vi "Is_Active_Call.vi"(5 "Enum":T1(ring), 6 "error in (no error)":errorcluster, 7 "Floor":i32, 8 "Elevator in":T3, 9 "Elevator Fleet in":T2) -> (0 "error out":errorcluster, 1 "Active Call?":bool, 2 "Elevator out":T3, 3 "Elevator Fleet out":T2)   [LabVIEW 2026]
uses:
  Controls/Elevator_Status.ctl
  Controls/Door_Status_Enum.ctl
  Controls/Occupy_Status.ctl
  Controls/Floor_Status.ctl
  Controls/Motion_Status_Enum.ctl
  Controls/Car_Calls_Status.ctl
  Controls/Hall_Calls_Status.ctl
  Controls/Elevator_Fleet.ctl
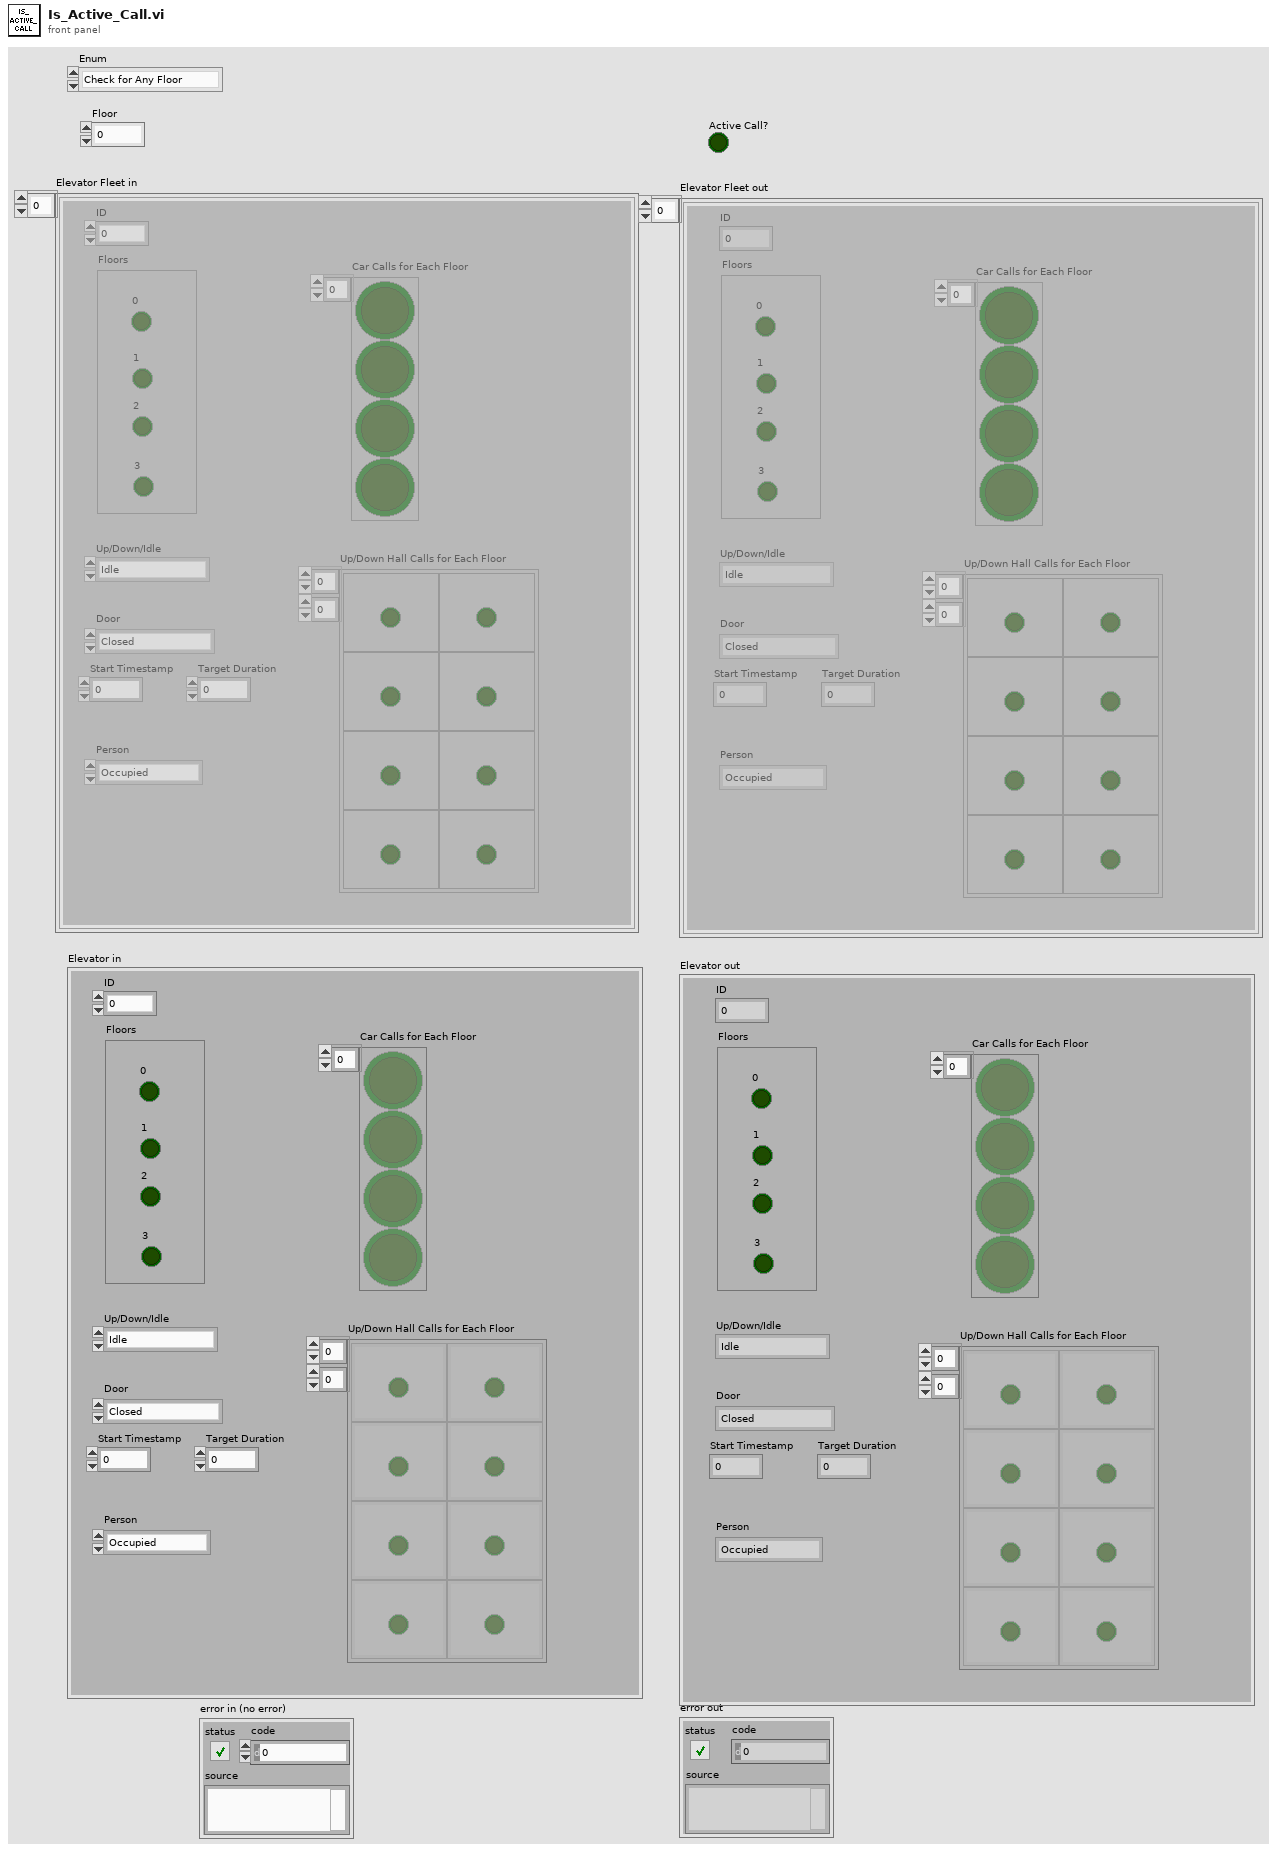
[diagram p1: front panel]
types:
  T1 = enum16{"Check for Any Floor", "Check for Specific Floor"}
  T2 = typedef "Elevator_Fleet.ctl" = T3[]
  T3 = typedef "Elevator_Status.ctl" = cluster{"Door":T4, "Person":T5, "Floors":T6, "Up/Down/Idle":T7, "Car Calls for Each Floor":T8, "Up/Down Hall Calls for Each Floor":T9, "ID":i32, "Start Timestamp":u32, "Target Duration":dbl}
  T4 = typedef "Door_Status_Enum.ctl" = enum16{"Closed", "Open", "Opening", "Closing"}
  T5 = typedef "Occupy_Status.ctl" = enum16{"Occupied", "Empty"}
  T6 = typedef "Floor_Status.ctl" = cluster{"0":bool, "1":bool, "2":bool, "3":bool}
  T7 = typedef "Motion_Status_Enum.ctl" = enum16{"Idle", "Up", "Down"}
  T8 = typedef "Car_Calls_Status.ctl" = bool[]
  T9 = typedef "Hall_Calls_Status.ctl" = cluster{bool}[][]
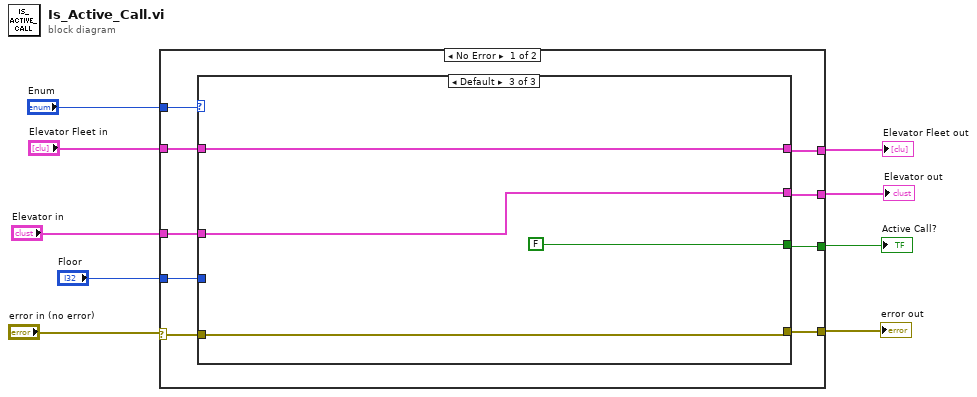
[diagram p0: block diagram]
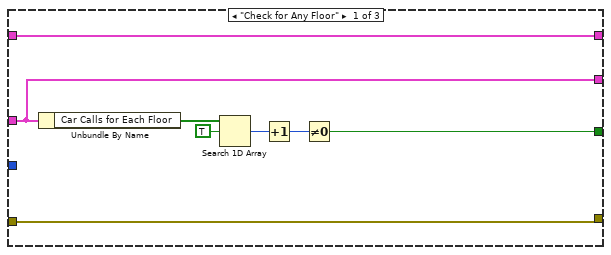
[diagram p2: hidden frame]
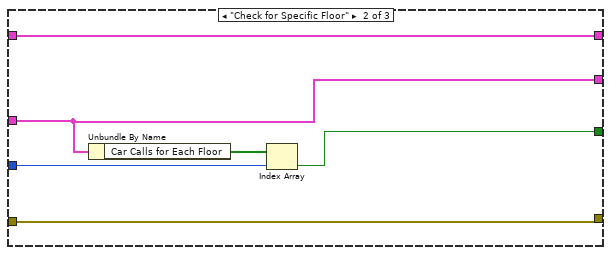
[diagram p3: hidden frame]
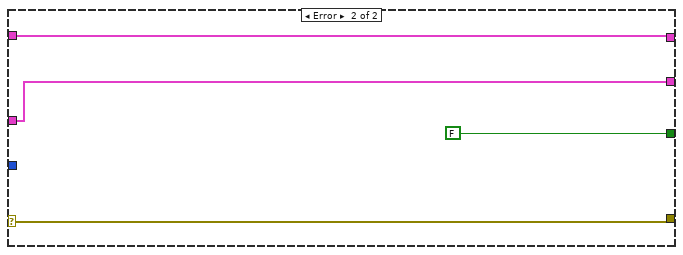
[diagram p4: hidden frame]
diagram:
  n1 = case shown="No Error" "error in (no error)" {
    selector: "error in (no error)" -> [w12 w38]
    tunnel: "Elevator in" -> [w18 w39]
    tunnel: [w17 FALSE] -> w8
    tunnel: [w16 w39] -> w7
    tunnel: "Elevator Fleet in" -> [w15 w40]
    tunnel: [w14 w40] -> w5
    tunnel: "Enum" -> [w13 _]
    tunnel: [w11 w38] -> w2
    tunnel: "Floor" -> [w10 _]
    frame No Error {
      n2 = case shown="Default" w13 {
        tunnel: w18 -> [w21 w30 w35]
        tunnel: [w22 w27 FALSE] -> w17
        tunnel: [w21 w30 w35] -> w16
        tunnel: w15 -> [w20 w31 w36]
        tunnel: [w20 w31 w36] -> w14
        tunnel: [w19 w32 w33] -> w11
        tunnel: w12 -> [w19 w32 w33]
        tunnel: w10 -> [_ w28 _]
        frame "Check for Any Floor" {
          n3 = Unbundle By Name(w21) -> ("Car Calls for Each Floor"=w26:T8)
          n4 = Search 1D Array(1D array=w26, element=TRUE) -> (index of element=w24:i32)  [unwired: 1 in]
          n5 = Increment(x=w24) -> (x+1=w23:i32)
          n6 = Not Equal To 0?(x=w23) -> (x != 0?=w22:bool)
        }
        frame "Check for Specific Floor" {
          n7 = Unbundle By Name(w30) -> ("Car Calls for Each Floor"=w29:T8)
          n8 = Index Array(array=w29, index=w28) -> (element=w27:bool)
        }
        frame Default {
        }
      }
    }
    frame Error {
    }
  }
  "Active Call?" <- w8
  "error out" <- w2
  "Elevator out" <- w7
  "Elevator Fleet out" <- w5
